vi "_DServerEventCreate.vi"(0 "error in":errorcluster) -> (1 "error out":errorcluster, 2 "dserver evt.":T1)   [LabVIEW 2014, in "tango.lvlib"]
uses:
  tango.lvlib
  Typedefs/_DServerClientRequest.ctl
  Typedefs/_DServerClientRequestType.ctl
  Typedefs/_DServerClientRequestData.ctl
  Typedefs/_GenericDataBuffer.ctl
  Typedefs/_DataType.ctl
panel:
  in  "tango client request":T2={"Request Id"=0, "Source Id"=0, "Request Type"=enum."UNKNOWN_REQUEST", "Device Class Name"="unspecified_cmd_or_attr_name", "Device Name"="unspecified/device/name", "Cmd or Attr Name"="unspecified_cmd_or_attr_name", "Client Request Data"={"write attribute value"={"dimx"=0, "dimy"=0, "data"=[], "data_type"=enum."UNKNOWN_DATA_TYPE"}, "exec. command argin"={"num data"=[], "str data"=[]}}}
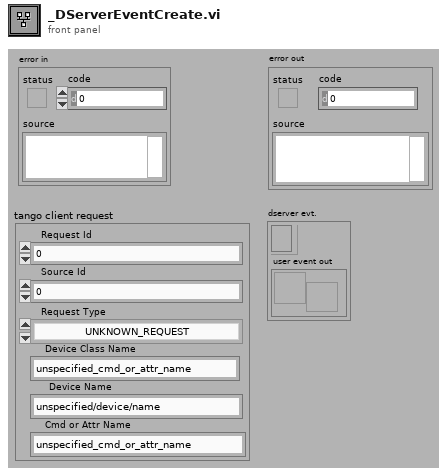
[diagram p1: front panel]
types:
  T1 = cluster{"event registration refnum":refnum<event-registration>, "user event out":refnum<user-event>}
  T2 = typedef "tango.lvlib/_DServerClientRequest.ctl" = cluster{"Request Id":u32, "Source Id":u32, "Request Type":T3, "Device Class Name":string, "Device Name":string, "Cmd or Attr Name":string, "Client Request Data":T4}
  T3 = typedef "tango.lvlib/_DServerClientRequestType.ctl" = enum16{"EXEC_CMD", "READ_ATTR", "WRITE_ATTR", "UNKNOWN_REQUEST"}
  T4 = typedef "tango.lvlib/_DServerClientRequestData.ctl" = cluster{"write attribute value":T5, "exec. command argin":cluster{"num data":u8[], "str data":string[]}}
  T5 = typedef "tango.lvlib/_GenericDataBuffer.ctl" = cluster{"dimx":u32, "dimy":u32, "data":u8[], "data_type":T6}
  T6 = typedef "tango.lvlib/_DataType.ctl" = enum16{"STATE_SCA", "STATE_SPE", "STATE_IMG", "STRING_SCA", "STRING_SPE", "STRING_IMG", "BOOL_SCA", "BOOL_SPE", "BOOL_IMG", "UCHAR_SCA", "UCHAR_SPE", "UCHAR_IMG", "SHORT_SCA", "SHORT_SPE", "SHORT_IMG", "USHORT_SCA", "USHORT_SPE", "USHORT_IMG", "LONG_SCA", "LONG_SPE", "LONG_IMG", "ULONG_SCA", "ULONG_SPE", "ULONG_IMG", "LONG64_SCA", "LONG64_SPE", "LONG64_IMG", "ULONG64_SCA", "ULONG64_SPE", "ULONG64_IMG", "FLOAT_SCA", "FLOAT_SPE", "FLOAT_IMG", "DOUBLE_SCA", "DOUBLE_SPE", "DOUBLE_IMG", "SCA_ENCODED", "SPE_ENCODED", "IMG_ENCODED", "UNKNOWN_DATA_TYPE"}
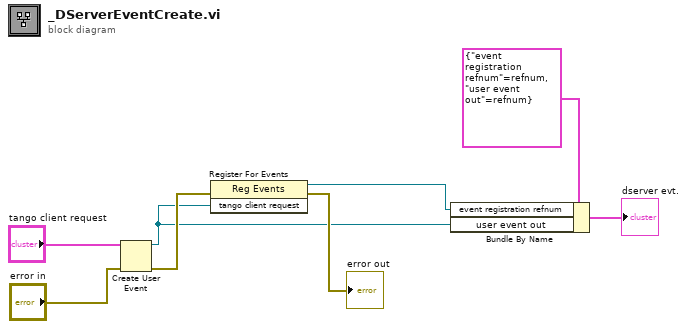
[diagram p0: block diagram]
diagram:
  n1 = Create User Event(user event datatype="tango client request", error in="error in") -> (user event=w2:refnum<user-event>, error out=w7:errorcluster)
  n2 = register-events(error in=w7, w2) -> (reference out=w4:refnum<event-registration>, error out=→"error out":errorcluster)  [unwired: 1 in]
  n3 = Bundle By Name(cluster=T1 {"event registration refnum"=refnum, "user event out"=refnum}, "event registration refnum"=w4, "user event out"=w2) -> (→"dserver evt.":T1)
